vi "ClassAttributes_ReadClassAttributes_6x8x6_Singleton.vi"(5 "error in (no error)":errorcluster) -> (19 "error out":errorcluster)   [LabVIEW 2016]
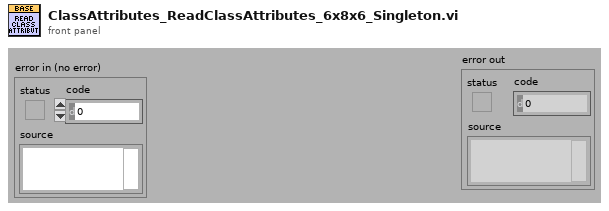
[diagram p1: front panel]
types:
  T1 = typedef "ClassAttributes_ClassAttributes.ctl" = cluster{"classAttribute1":bool}
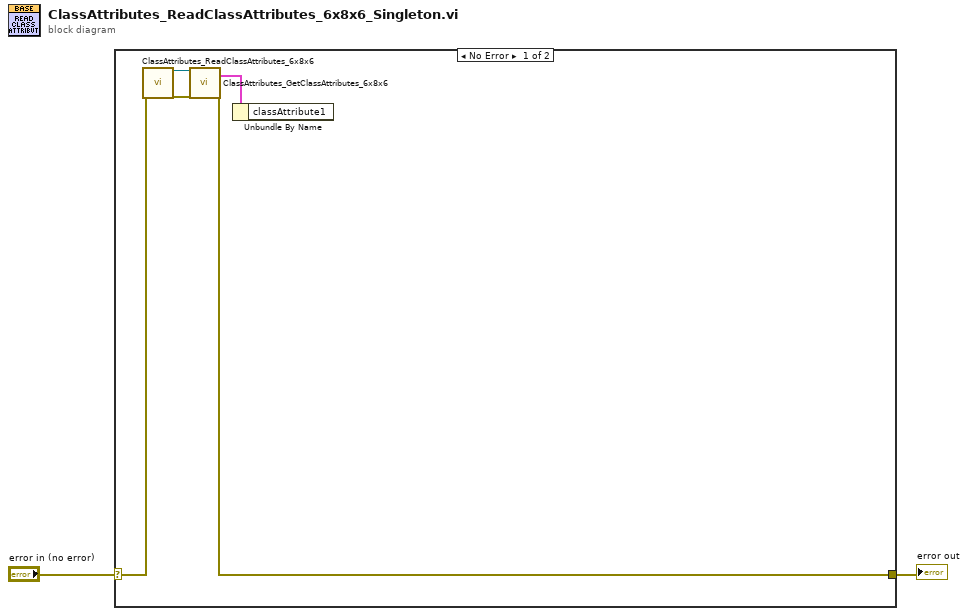
[diagram p0: block diagram]
diagram:
  n1 = case shown="No Error" "error in (no error)" {
    selector: "error in (no error)" -> [w3 w8]
    tunnel: [w6 w8] -> w1
    frame No Error {
      n2 = call <resource>:"ClassAttributes_ReadClassAttributes_6x8x6.vi"("error in (no error)"=w3) -> ("reference out"=w5:refnum<class>, "error out"=w4:errorcluster)  [unwired: 17 in]
      n3 = call <resource>:"ClassAttributes_GetClassAttributes_6x8x6.vi"("reference in"=w5, "error in (no error)"=w4) -> ("Class attribute"=w7:T1, "error out"=w6:errorcluster)  [unwired: 14 in, 2 out]
      n4 = Unbundle By Name(w7) -> ()  [unwired: 1 out]
    }
    frame Error {
    }
  }
  "error out" <- w1
